vi "Save_USB_Address_Config_File.vi"(0 "App Path":path, 1 "USB DAQ Address":i32) -> ()   [LabVIEW 2011]
doc: "This VI is called from \"Start USB\". This will change the address stored in \"USB_DAQ.ini\" if the user chooses a new address in the \"Start USB\" VI. It will not edit any other items in the USB_DAQ.ini file."
uses:
  INA231/Global 1.vi
  <vilib>/Utility/config.llb/Write Key (I32).vi
  <vilib>/Utility/config.llb/NI_LVConfig.lvlib
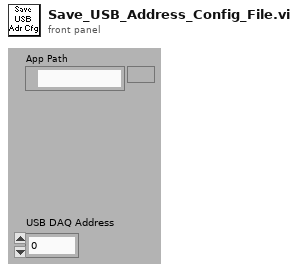
[diagram p1: front panel]
types:
  T1 = typedef "NI_LVConfig.lvlib/Config Data RefNum.ctl" = refnum<k1>
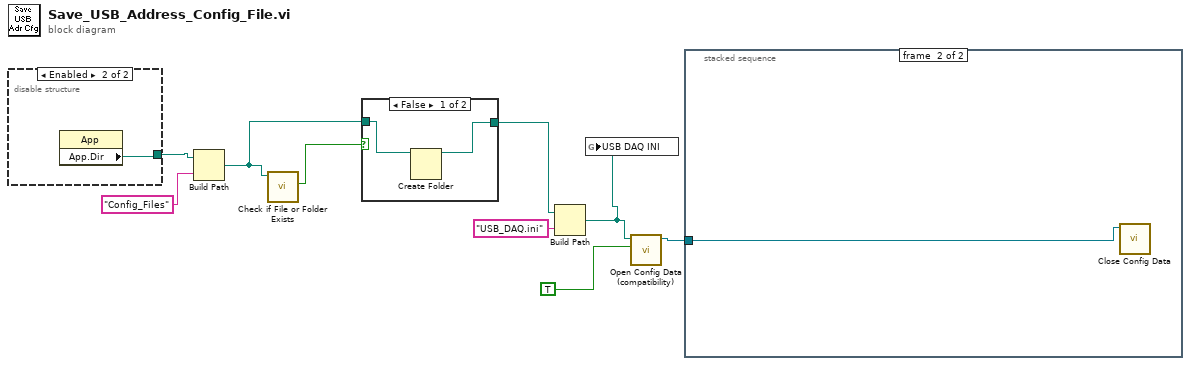
[diagram p0: block diagram]
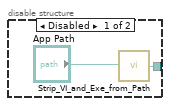
[diagram p2: hidden frame]
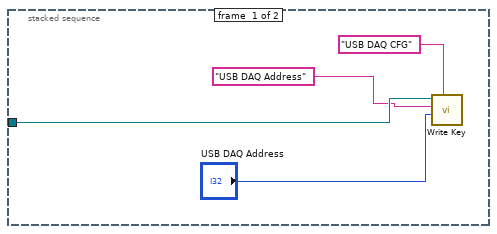
[diagram p4: hidden frame]
diagram:
  n1 = disable-structure shown="Enabled" {
    disable-tunnel: [w10 w12] -> w2
    frame Disabled {
      n2 = call "Strip_VI_and_Exe_from_Path.vi"("App Path"="App Path") -> ("App Path out"=w10:path)
    }
    frame Enabled {
      n3 = property class="App"() -> ("App.Dir"=w12:path)  [unwired: 2 in, 2 out]
    }
  }
  n4 = Build Path(base path=w2, name or relative path="Config_Files") -> (appended path=w4:path)
  n5 = call <vilib>:"Check if File or Folder Exists.vi"("path"=w4) -> ("file or folder exists?"=w5:bool)  [unwired: 8 in, 2 out]
  n6 = case shown="False" w5 {
    tunnel: w4 -> [w14 w15]
    tunnel: [w13 w15] -> w3
    frame False {
      n7 = Create Folder(path (use dialog)=w14) -> (created path=w13:path)  [unwired: 2 in, 2 out]
    }
    frame True {
    }
  }
  n8 = Build Path(base path=w3, name or relative path="USB_DAQ.ini") -> (appended path=w1:path)
  n9 = global write "Global 1.vi" "USB DAQ INI"(w1) -> ()
  n10 = call <vilib>:"Open Config Data (compatibility).vi"("create file if necessary (T)"=TRUE ("create file if necessary? (T)"), "configuration file path"=w1) -> ("refnum"=w7:T1)  [unwired: 7 in, 2 out]
  n11 = stacked-sequence {
    tunnel: w7 -> [w19 w20]
    frame #0 {
      n12 = call-poly <vilib>:"Write Key.vi"("section"="USB DAQ CFG", "value"="USB DAQ Address", "key"="USB DAQ Address" ("section"), "refnum"=w19) -> ()  [unwired: 5 in, 3 out]
    }
    frame #1 {
      n13 = call <vilib>:"Close Config Data.vi"("refnum"=w20) -> ()  [unwired: 9 in, 2 out]
    }
  }
